vi "Open Connection to Tags.vi"(7 "Publish":bool, 8 "error in (no error)":errorcluster, 10 "data type":T1 caption="Data Type", 11 "Tag.Paths":string[](array[string])) -> (0 "error out":errorcluster, 3 "SysLink.Refs":refnum<class "NI Skyline Tag.lvclass">[](array[class]))   [LabVIEW 2019, in "Data Publishing Service.lvlib"]
uses:
  Data Publishing Service.lvlib
  <vilib>/Skyline/Tag/Wrapper/Wrapper_class/NI Skyline Tag.lvclass
  <vilib>/Skyline/Tag/Shared/typedefs/DataType.ctl
  <vilib>/Skyline/Tag/Wrapper/Wrapper HTTP_class/NI Skyline Tag HTTP.lvclass
  <vilib>/Skyline/Tag/Shared/NI Skyline Tag.lvlib
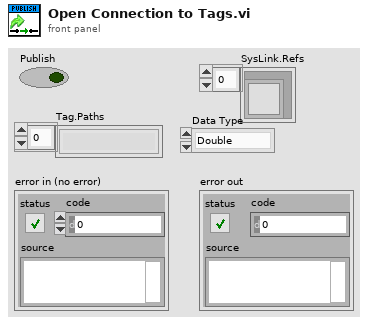
[diagram p1: front panel]
types:
  T1 = typedef "NI Skyline Tag.lvlib/DataType.ctl" = enum32{"Double", "I32", "String", "Boolean", "U64", "Timestamp"}
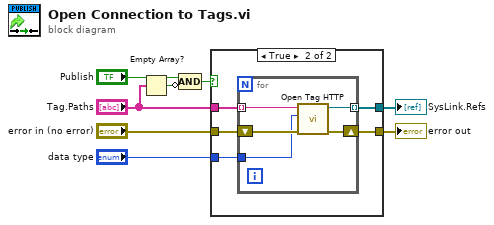
[diagram p0: block diagram]
diagram:
  n1 = Empty Array?(array="Tag.Paths") -> (empty?=w7:bool)
  n2 = Compound Arithmetic op=AND("Publish", invert w7) -> (w8:bool)
  n3 = case shown="True" w8 {
    tunnel: "Tag.Paths" -> [_ w14]
    tunnel: "error in (no error)" -> [w9 w13]
    tunnel: [w9 w12] -> w4
    tunnel: [_ w11] -> w5
    tunnel: "data type" -> [_ w10]
    frame False {
    }
    frame True {
      n4 = for {
        shift-right: [w18] -> w12
        shift-left: w13 -> [w19]
        tunnel: w14 -> [w17] mode=indexing
        tunnel: [w16] -> w11 mode=indexing
        tunnel: w10 -> [w15]
        n5 = call <vilib>:"Open Tag HTTP.vi"("error in (no error)"=w19, "Data Type"=w15, "path"=w17) -> ("error out"=w18:errorcluster, "tag"=w16:refnum<class "NI Skyline Tag.lvclass">)  [unwired: 7 in]
      }
    }
  }
  "SysLink.Refs" <- w5
  "error out" <- w4
